vi "Set Section CD Item Property Values.vi"(8 "error in (no error)":errorcluster, 11 "CD Parameter Manager in":refnum<class "CD Parameter Manager.lvclass">) -> (0 "error out":errorcluster, 3 "CD Parameter Manager out":refnum<class "CD Parameter Manager.lvclass">)   [LabVIEW 2016, in "CD Parameter Manager API.lvlib" / "CD Parameter Manager.lvclass"]
uses:
  CD Parameter Manager.lvclass
  Parameter Class/Parameter.lvclass
panel:
  in  "Group name":string
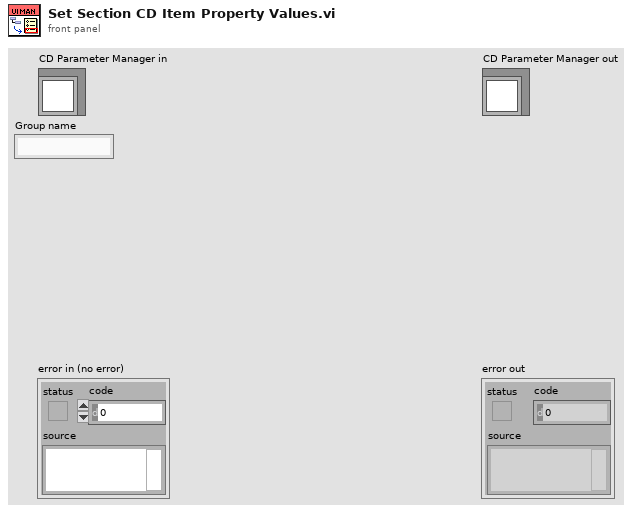
[diagram p1: front panel]
types:
  T1 = cluster{"Group name":string, "Controls":refnum<class "Parameter.lvclass">[]}[]
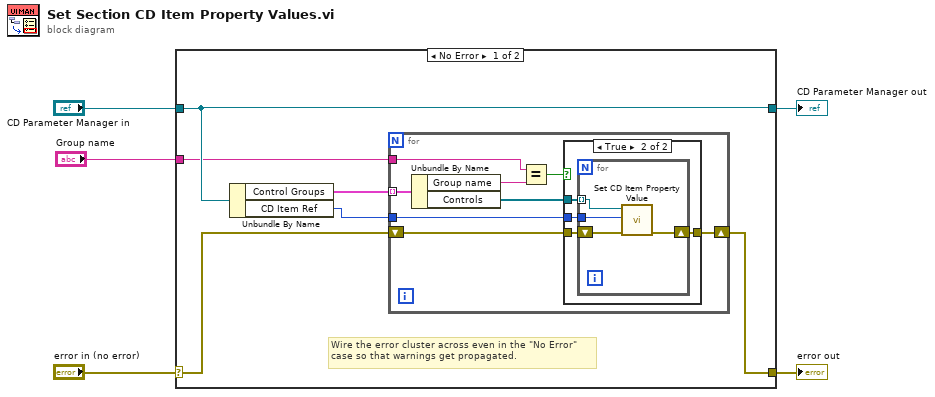
[diagram p0: block diagram]
diagram:
  n1 = case shown="No Error" "error in (no error)" {
    selector: "error in (no error)" -> [w8 w30]
    tunnel: [w7 w30] -> w4
    tunnel: [w9 w29] -> w2
    tunnel: "CD Parameter Manager in" -> [w9 w29]
    tunnel: "Group name" -> [w6 _]
    frame No Error {
      # "Wire the error cluster across even in the \"No Error\"\ncase so that warnings get propagated."
      n2 = Unbundle By Name(w9) -> ("Control Groups"=w11:T1, "CD Item Ref"=w10:u64)
      n3 = for {
        tunnel: w11 -> [w17] mode=indexing
        tunnel: w10 -> [w15]
        shift-right: [w18] -> w7
        shift-left: w8 -> [w19]
        tunnel: w6 -> [w13]
        n4 = Unbundle By Name(w17) -> ("Group name"=w14:string, "Controls"=w16:refnum<class "Parameter.lvclass">[])
        n5 = Equal?(x=w13, y=w14) -> (x = y?=w12:bool)
        n6 = case shown="True" w12 {
          tunnel: w19 -> [w20 w24]
          tunnel: [w20 w23] -> w18
          tunnel: w16 -> [_ w22]
          tunnel: w15 -> [_ w21]
          frame False {
          }
          frame True {
            n7 = for {
              tunnel: w21 -> [w26]
              shift-right: [w27] -> w23
              shift-left: w24 -> [w28]
              tunnel: w22 -> [w25] mode=indexing
              n8 = call-dynamic "Set CD Item Property Value.vi"("error in (no error)"=w28, "CD Item Ref in"=w26, "Parameter in"=w25) -> ("error out"=w27:errorcluster)  [unwired: 7 in, 1 out]
            }
          }
        }
      }
    }
    frame Error {
    }
  }
  "error out" <- w4
  "CD Parameter Manager out" <- w2
